vi "From Variant.vi"(0 "Obj in":refnum<class "FSM.Edge.lvclass">, 7 "Variant":variant, 9 "Prefix":string, 11 "error in (no error)":errorcluster) -> (4 "Obj out":refnum<class "FSM.Edge.lvclass">, 15 "error out":errorcluster)   [LabVIEW 2020, in "FSM.Edge.lvclass"]
uses:
  FSM.Edge.lvclass
  FSM.Edge.lvclass/FSM.Edge.ctl
  epl-vi-lib/Koop/KObject Class/KObject.lvclass
  FSM.Label/FSM.Label.lvclass
  FSM.EdgeEnd/FSM.EdgeEnd.lvclass
  FSM.Annotation/FSM.Annotation.lvclass
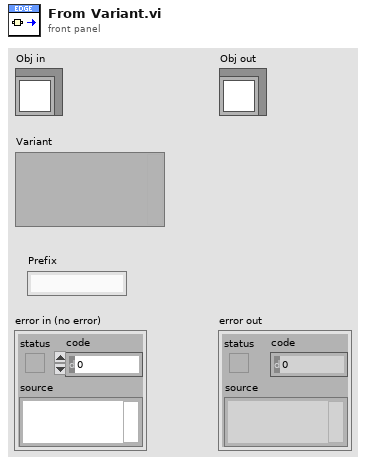
[diagram p1: front panel]
types:
  T1 = typedef "FSM.Edge.lvclass/Serialized.ctl" = cluster{"Label":refnum<class "FSM.Label.lvclass">, "SourceName":string, "TargetName":string, "Points":cluster{"x":i16, "y":i16}[], "Color":u32, "Style":enum32{"Solid", "Dash", "Dot", "DashDot", "DashDotDot"}, "SourceEnd":refnum<class "FSM.EdgeEnd.lvclass">, "TargetEnd":refnum<class "FSM.EdgeEnd.lvclass">, "Type":string, "Annotations":refnum<class "FSM.Annotation.lvclass">}
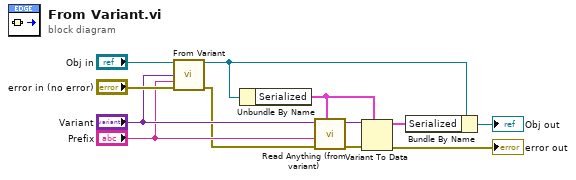
[diagram p0: block diagram]
diagram:
  n1 = call-parent "From Variant.vi"("KObject in"="Obj in", "Variant"="Variant", "Prefix"="Prefix", "error in (no error)"="error in (no error)") -> ("KObject out"=w3:refnum<class "FSM.Edge.lvclass">, "error out"=w4:errorcluster)  [unwired: 10 in]
  n2 = Unbundle By Name(w3) -> ("Serialized"=w8:T1)
  n3 = call "Read Anything (from variant).vi"("Type of Anything"=w8, "Error In"=w4, "Prefix"="Prefix", "Variant Database"="Variant") -> ("Error Out"=w9:errorcluster, "Anything"=w10:variant)  [unwired: 5 in, 1 out]
  n4 = Variant To Data(error in=w9, type=w8, Variant=w10) -> (data=w7:T1, error out=→"error out":errorcluster)
  n5 = Bundle By Name(cluster=w3, "Serialized"=w7) -> (→"Obj out":refnum<class "FSM.Edge.lvclass">)
